vi "Osc_gen_stp.vi"() -> ()   [LabVIEW 2018]
uses:
  <vilib>/LabVIEW Interface for Arduino/Type Defs/Board Type.ctl
  <vilib>/LabVIEW Interface for Arduino/Type Defs/Connection Type.ctl
  <instrlib>/LeCroy Wave Series/Public/Data/Read Single Waveform.vi
  <vilib>/LabVIEW Interface for Arduino/LabVIEW Interface for Arduino.lvlib
  <instrlib>/LeCroy Wave Series/LeCroy Wave Series.lvlib
panel:
  out "relative seconds 2":dbl format="%_19f"
  out "relative seconds":dbl format="%_19f"
  in  "Tab Control":enum32{"Page 3", "Page 1", "Page 2"}(tab)
  in  "VISA resource":refnum<visa-resource-name>
  in  "Board Type (Uno)":T1
  in  "error in":errorcluster
  in  "Stepper #":u8
  in  "Control Method":u8(ring)=1 items=["2 Wire (Pulse & Direction)"=1, "2 Wire"=2, "4 Wire"=4, "EasyDriver"=6, "AF Motor Shield (Stepper 1 & 2 Only)"=5]
  in  "Steps for one rotation":i16
  in  "Set Speed (Steps per Second)":i16=100
  out "Steps Remaining?":bool
  in  "Step Size":i16
  out "Step Angle":dbl
  in  "Baud Rate":u32=115200
  out "Iteration #":i32
  out "Steps Remaining? 2":bool
  in  "# of translation Steps":i16
  in  "# of Steps to Move":i16
  out "Iteration #2":i32
  out "error out":errorcluster
  in  "VISA Refnum in":refnum<visa-resource-name>
  in  "Channel (1:Channel 1)":i32(ring)=1 items=["Channel 1"=1, "Channel 2"=2]
  in  "Enable Output (T: Enable)":bool=TRUE
  in  "Amplitude (1.0 Vpp)":dbl=1.0 format="%#.3f"
  in  "Frequency (1000 Hz)":dbl=1000.0 format="%#.6g"
  in  "DC Offset (0.00 V) in":dbl
  in  "Waveform Function (0: Sine) in":u16(ring) items=["Sine", "Square", "Ramp", "DC", "Pulse", "Arb"]
  in  "Phase (0.0 degrees)":dbl=0.002 min=-360.0 max=360.0 format="%#.1g"
  in  "True To \ngenerate\n pulse":bool
  out "VISA resource name out":refnum<visa-resource-name>
  out "error out 2":errorcluster
  out "Output Filename":path
  out "error out 3":errorcluster
  in  "format string":string
  out "Output Directory":path
  in  "File Directory":path
  in  "Filename":string
  in  "Rise (20 ns)":dbl=2e-08 format="%#.3g"
  in  "Delay (0.00 s)":dbl min=-1000000.0 max=1000000.0
  in  "Fall (20 ns)":dbl=2e-08 format="%#.3g"
  in  "Duty (20%)":dbl=20.0 min=0.0001 max=100.0 format="%.4g"
  out ".not. x?":bool
  in  "stop":bool
  out "Waveform Data":waveform(dbl)(graph)
  in  "Timeout (10000 ms)":u32=10000
  in  "Source (0: Channel 1)":u16(ring) items=["Channel 1", "Channel 2", "Channel 3", "Channel 4", "Memory 1", "Memory 2", "Memory 3", "Memory 4", "Function 1", "Function 2", "Function 3", "Function 4", "Function 5", "Function 6", "Function 7", "Function 8"]
  in  "Perform Auto Setup?":bool
  in  "Reset Scope?":bool
  in  "VISA resource name":refnum<visa-resource-name>
  out "Saved filename":string
  in  "Save Files in Directory":string="D:\\Automation\\Data"
  # "Set PULSE parameters"
  # "In the oscilloscope memory"
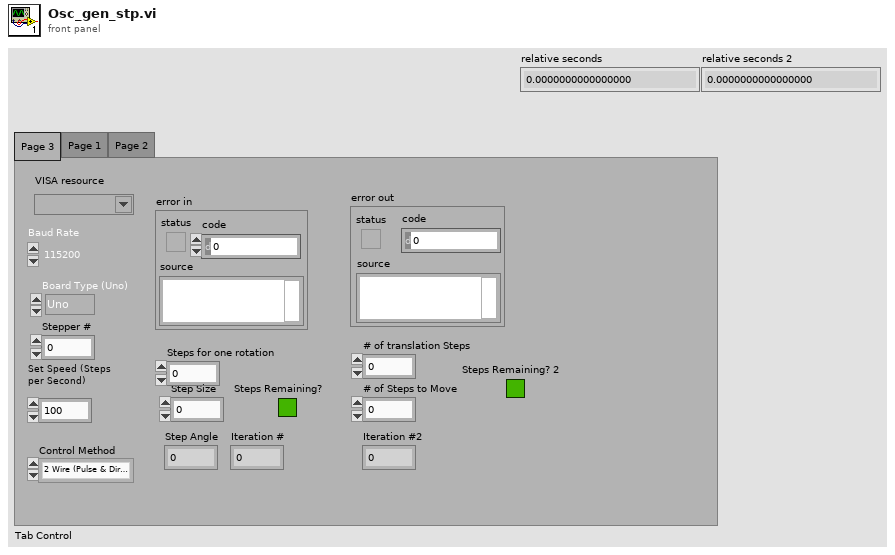
[diagram p1: front panel]
types:
  T1 = typedef "LabVIEW Interface for Arduino.lvlib/Board Type.ctl" = enum16{"Uno", "Dimuelanove w/Atmega 328", "Mega 2560"}
  T2 = typedef "LabVIEW Interface for Arduino.lvlib/Connection Type.ctl" = enum8{"USB / Serial", "XBEE", "BlueSmirf (Bluetooth)"}
  T3 = typedef "LabVIEW Interface for Arduino.lvlib/Arduino Resource.ctl" = cluster{"VISA resource":refnum<visa-resource-name>, "Board Type":T1, "Connection Type":enum8{"USB / Serial"}, "Bytes Per Packet (15)":u8}
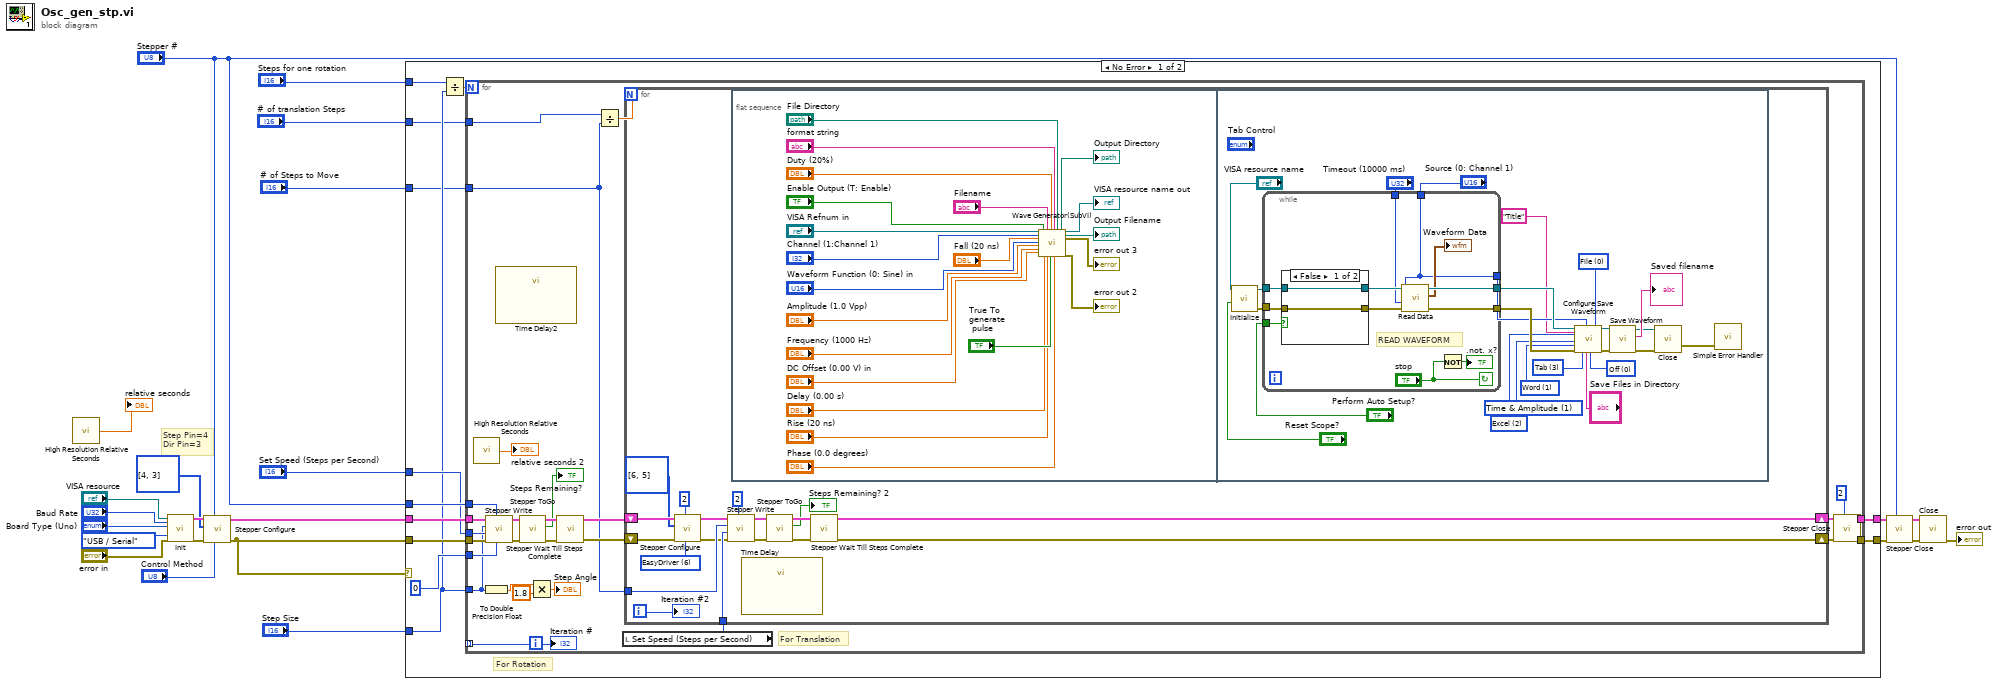
[diagram p0: block diagram]
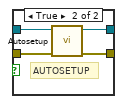
[diagram p2: hidden frame]
diagram:
  # "Step Pin=4\nDir Pin=3"
  n1 = call <vilib>:"High Resolution Relative Seconds.vi"() -> ("relative seconds"=→"relative seconds":dbl)
  n2 = call <vilib>:"Init.vi"("VISA resource"="VISA resource", "Baud Rate (115200)"="Baud Rate", "Board Type (Uno)"="Board Type (Uno)", "Connection Type (USB/Serial)"=Connection_Type."USB / Serial", "error in"="error in") -> ("Arduino Resource"=w20:T3, "error out"=w19:errorcluster)  [unwired: 13 in]
  n3 = call <vilib>:"Stepper Configure.vi"("Control Method"="Control Method", "Stepper #"="Stepper #", "error in"=w19, "Stepper Pins"=u8[] [4, 3], "Arduino Resource"=w20) -> ("error out"=w2:errorcluster, "Arduino Resource Out"=w10:T3)  [unwired: 5 in]
  n4 = case shown="No Error" w2 {
    tunnel: [w35 w145] -> w13
    tunnel: [w34 w144] -> w12
    tunnel: "Stepper #" -> [w33 _]
    tunnel: w2 -> [w32 w145]
    tunnel: w10 -> [w31 w144]
    tunnel: "Set Speed (Steps per Second)" -> [w28 _]
    tunnel: "Step Size" -> [w27 _]
    tunnel: "# of Steps to Move" -> [w26 _]
    tunnel: "Steps for one rotation" -> [w25 _]
    tunnel: "# of translation Steps" -> [w24 _]
    frame No Error {
      # "For Rotation"
      n5 = Divide(x=w25, y=w27) -> (x/y=w29:dbl)
      n6 = for {
        N: w29 -> [_]
        tunnel: [w42] -> w35
        tunnel: [w40] -> w34
        tunnel: i16 0 ("Acceleration") -> [w59]
        tunnel: w33 -> [w58]
        tunnel: w32 -> [w57]
        tunnel: w28 -> [w56]
        tunnel: w31 -> [w55]
        tunnel: [w49] -> _ mode=indexing
        tunnel: w27 -> [w48]
        tunnel: w26 -> [w38]
        tunnel: w24 -> [w37]
        i -> [w49]
        # "For Translation"
        n7 = call <vilib>:"High Resolution Relative Seconds.vi"() -> ("relative seconds"=→"relative seconds 2":dbl)
        n8 = To Double Precision Float(number=w48) -> (double precision float=w51:dbl)
        n9 = call <vilib>:"Stepper Write.vi"("Set Acceleration (0 to disable)"=w59, "Stepper #"=w58, "error in"=w57, "Set Speed (Steps per Second)"=w56, "# of Steps to Move"=w48, "Arduino Resource"=w55) -> ("error out"=w54:errorcluster, "Arduino Resource Out"=w53:T3)  [unwired: 4 in]
        n10 = call "Time Delay2"() -> ()  [unwired: 11 in, 1 out]
        n11 = call <vilib>:"Stepper ToGo.vi"("error in"=w54, "Arduino Resource"=w53) -> ("error out"=w62:errorcluster, "Steps Remaining?"=→"Steps Remaining?":bool, "Arduino Resource Out"=w61:T3)  [unwired: 6 in, 1 out]
        n12 = Multiply(x=w51, y=1.8) -> (x*y=→"Step Angle":dbl)
        n13 = call <vilib>:"Stepper Wait Till Steps Complete.vi"("error in"=w62, "Arduino Resource In"=w61) -> ("error out"=w47:errorcluster, "Arduino Resource Out"=w46:T3)  [unwired: 8 in]
        n14 = Divide(x=w37, y=w38) -> (x/y=w45:dbl)
        n15 = local read "Set Speed (Steps per Second)"() -> (w44:i16)
        n16 = for {
          N: w45 -> [_]
          shift-right: [w75] -> w41
          shift-left: w46 -> [w70]
          shift-right: [w74] -> w43
          shift-left: w47 -> [w68]
          tunnel: w38 -> [w72]
          tunnel: w44 -> [w71]
          i -> [w63]
          w64 = u8 6 items=["2 Wire (Pulse & Direction)"=1, "2 Wire"=2, "4 Wire"=4, "EasyDriver"=6, "AF Motor Shield (Stepper 1 & 2 Only)"=5] ("Control Method")
          n17 = call <vilib>:"Stepper Configure.vi"("Control Method"=w64, "Stepper #"=u8 2, "error in"=w68, "Stepper Pins"=u8[] [6, 5], "Arduino Resource"=w70) -> ("error out"=w67:errorcluster, "Arduino Resource Out"=w69:T3)  [unwired: 5 in]
          n18 = call <vilib>:"Stepper Write.vi"("Stepper #"=u8 2, "error in"=w67, "Set Speed (Steps per Second)"=w71, "# of Steps to Move"=w72, "Arduino Resource"=w69) -> ("error out"=w77:errorcluster, "Arduino Resource Out"=w76:T3)  [unwired: 5 in]
          n19 = flat-sequence {
            frame #0 {
              n20 = call "Wave Generator(SubVI).vi"("VISA Refnum in"="VISA Refnum in", "Channel (1:Channel 1)"="Channel (1:Channel 1)", "Fall (20 ns)"="Fall (20 ns)", "Waveform Function (0: Sine) in"="Waveform Function (0: Sine) in", "Amplitude (1.0 Vpp)"="Amplitude (1.0 Vpp)", "Frequency (1000 Hz)"="Frequency (1000 Hz)", "DC Offset (0.00 V) in"="DC Offset (0.00 V) in", "Enable Output (T: Enable)"="Enable Output (T: Enable)", "Delay (0.00 s)"="Delay (0.00 s)", "Filename"="Filename", "Rise (20 ns)"="Rise (20 ns)", "Duty (20%)"="Duty (20%)", "True To \ngenerate\n pulse"="True To \ngenerate\n pulse", "format string"="format string", "Phase (0.0 degrees)"="Phase (0.0 degrees)", "File Directory"="File Directory") -> ("Output Directory"=→"Output Directory":path, "VISA Refnum out"=→"VISA resource name out":refnum<visa-resource-name>, "Output Filename"=→"Output Filename":path, "error out 2"=→"error out 3":errorcluster, "error out"=→"error out 2":errorcluster)  [unwired: 7 in]
            }
            frame #1 {
              w108 = u16 3 items=["Comma", "Space", "Semicolon", "Tab"] ("Delimiter (  0:Comma)")
              w109 = u16 0 items=["Off", "Wrap", "Fill"] ("Auto Save (0:Off")
              w110 = u16 1 items=["Byte", "Word", "Auto"] ("BinarySubFormat (1: Word)")
              w112 = u16 1 items=["Amplitude Only", "Time & Amplitude", "With Header"] ("SubFormat (1: Time & Amplitude)")
              w113 = u16 2 items=["Binary", "ASCII", "Excel", "MATLAB", "MathCad", "WaveML"] ("Format (0: Binary)")
              w114 = u16 0 items=["File", "M1", "M2", "M3", "M4"] ("Destination (0:File)")
              n21 = call <instrlib>:"Initialize.vi"("Reset? (T: Yes)"="Reset Scope?", "VISA resource name"="VISA resource name") -> ("error out"=w122:errorcluster, "VISA resource name out"=w123:refnum<visa-resource-name>)  [unwired: 8 in]
              n22 = while {
                tunnel: [w135] -> w116
                tunnel: [w134] -> w117
                tunnel: "Perform Auto Setup?" -> [w133]
                tunnel: "Source (0: Channel 1)" -> [w126]
                tunnel: w122 -> [w132]
                tunnel: w123 -> [w131]
                tunnel: "Timeout (10000 ms)" -> [w130]
                tunnel: [w126] -> w115
                stop <- "stop" continue-if-true
                # "READ WAVEFORM"
                n23 = case shown="False" w133 {
                  tunnel: w132 -> [w138 w143]
                  tunnel: w131 -> [w139 w142]
                  tunnel: [w139 w141] -> w137
                  tunnel: [w138 w140] -> w136
                  frame False {
                  }
                  frame True {
                    # "AUTOSETUP"
                    n24 = call <instrlib>:"Autosetup.vi"("error in (no error)"=w143, "VISA resource name"=w142) -> ("error out"=w140:errorcluster, "VISA resource name out"=w141:refnum<visa-resource-name>)  [unwired: 8 in]
                  }
                }
                n25 = call-poly <instrlib>:"Read Data.vi"("error in (no error)"=w136, "Timeout (10000 ms)"=w130, "Source (0: Channel 1)"=w126, "VISA resource name"=w137) -> ("error out"=w135:errorcluster, "Waveform Data"=→"Waveform Data":waveform(dbl), "VISA resource name out"=w134:refnum<visa-resource-name>)  [unwired: 5 in]
                n26 = Not(x="stop") -> (.not. x?=→".not. x?":bool)
              }
              n27 = call <instrlib>:"Configure Save Waveform.vi"("VISA resource name"=w117, "Trace Title (Title)"="Title", "Format (0: Binary)"=w113, "SubFormat (1: Time & Amplitude)"=w112, "BinarySubFormat (1: Word)"=w110, "error in (no error)"=w116, "Delimiter (  0:Comma)"=w108, "Source (0: Channel 1)"=w115, "Save Files in Directory (D:\\Waveforms)"="Save Files in Directory", "Auto Save (0:Off"=w109, "Destination (0:File)"=w114) -> ("VISA resource name out"=w106:refnum<visa-resource-name>, "error out"=w105:errorcluster)  [unwired: 7 in]
              n28 = call <instrlib>:"Save Waveform.vi"("error in (no error)"=w105, "VISA resource name"=w106) -> ("error out"=w102:errorcluster, "Saved filename"=→"Saved filename":string, "VISA resource name out"=w103:refnum<visa-resource-name>)  [unwired: 7 in]
              n29 = call <vilib>:"Close.vi"("error in (no error)"=w102, "VISA resource name"=w103) -> ("error out"=w125:errorcluster)  [unwired: 9 in]
              n30 = call <vilib>:"Simple Error Handler.vi"("error in (no error)"=w125) -> ()  [unwired: 4 in, 5 out]
            }
          }
          n31 = call "Time Delay"() -> ()  [unwired: 11 in, 1 out]
          n32 = call <vilib>:"Stepper ToGo.vi"("error in"=w77, "Arduino Resource"=w76) -> ("error out"=w80:errorcluster, "Steps Remaining?"=→"Steps Remaining? 2":bool, "Arduino Resource Out"=w79:T3)  [unwired: 6 in, 1 out]
          n33 = call <vilib>:"Stepper Wait Till Steps Complete.vi"("error in"=w80, "Arduino Resource In"=w79) -> ("error out"=w74:errorcluster, "Arduino Resource Out"=w75:T3)  [unwired: 8 in]
          "Iteration #2" <- w63
        }
        n34 = call <vilib>:"Stepper Close.vi"("Stepper #"=u8 2, "error in"=w43, "Arduino Resource"=w41) -> ("error out"=w42:errorcluster, "Arduino Resource Out"=w40:T3)  [unwired: 7 in]
        "Iteration #" <- w49
      }
    }
    frame Error {
    }
  }
  n35 = call <vilib>:"Stepper Close.vi"("Stepper #"="Stepper #", "error in"=w13, "Arduino Resource"=w12) -> ("error out"=w14:errorcluster, "Arduino Resource Out"=w15:T3)  [unwired: 7 in]
  n36 = call <vilib>:"Close.vi"("Arduino Resource"=w15, "error in"=w14) -> ("error out"=→"error out":errorcluster)  [unwired: 13 in]
